vi "Configure_Voltage.vi"(8 "error in (no error)":errorcluster, 10 "DC_Voltage_Configuration":variant, 11 "NI-DMM in":refnum<class "NI-DCPower.lvclass">) -> (0 "error out":errorcluster, 3 "NI-DMM out":refnum<class "NI-DCPower.lvclass">)   [LabVIEW 2020, in "NI-DCPower.lvclass"]
uses:
  NI-DCPower.lvclass
  C:/Program Files/National Instruments/LabVIEW 2020/vi.lib/MeasurementLink/MeasurementLink Instrument/ISession Factory/ISession Factory.lvclass
  Typedefs/Configure_Parameters.ctl
  <vilib>/MeasurementLink/MeasurementLink Session Management V1/Session Reservation/Pin Type.ctl
  Typedefs/connection with session.ctl
  <vilib>/MeasurementLink/MeasurementLink Session Management V1/Session Reservation/Connection.ctl
  <instrlib>/niDCPower/nidcpower.llb/niDCPower Source Mode.ctl
  f01df658-2e31-4a97-abfd-bc2b634ba6ad.vi
  <vilib>/MeasurementLink/MeasurementLink Session Management V1/Session Reservation/Get Connections Impl.vi
  <vilib>/MeasurementLink/MeasurementLink Session Management V1/Session Reservation/Session Reservation.lvclass
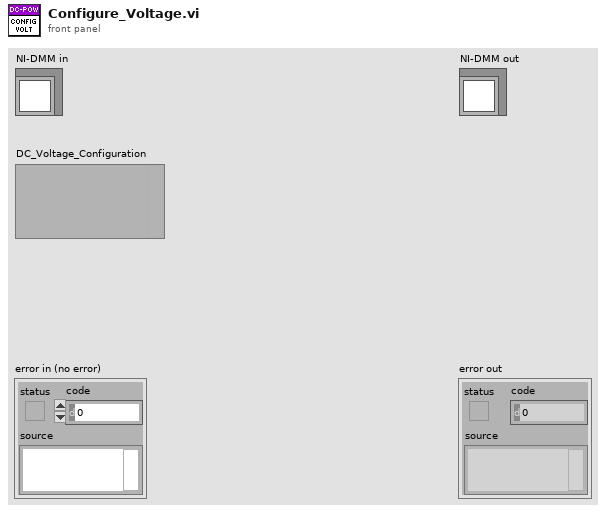
[diagram p1: front panel]
types:
  T1 = typedef "NI-DCPower.lvclass/connection with session.ctl" = cluster{"connection":T2, "session":refnum<k15>}
  T2 = typedef "MeasurementLink Session Management V1.lvlib/Session Reservation.lvclass/Connection.ctl" = cluster{"pin or relay name":string, "site":i32, "instrument type id":string, "channel":string}
  T3 = typedef "MeasurementLink Session Management V1.lvlib/Session Reservation.lvclass/Pin Type.ctl" = enum16{"DUT and System Pins", "System Pins"}
  T4 = typedef "NI-DCPower.lvclass/Configure_Parameters.ctl" = cluster{"pin name":string[], "Range":dbl, "Measurement Type":enum32{"DC Volts", "AC Volts", "DC Current", "AC Current", "2-wire Resistance", "4-wire Resistance", "Diode", "Frequency", "Period", "AC Volts DC Coupled", "Capacitance", "Inductance", "Temperature"}, "Resolution in Digits":enum32{"3 1/2", "4 1/2", "5 1/2", "6 1/2", "7 1/2"}}
  T5 = enum32{"DC Volts", "AC Volts", "DC Current", "AC Current", "2-wire Resistance", "4-wire Resistance", "Diode", "Frequency", "Period", "AC Volts DC Coupled", "Capacitance", "Inductance", "Temperature"}
  T6 = typedef "niDCPower Source Mode.ctl" = i32
  T7 = typedef "niDCPower Output Function.ctl" = i32
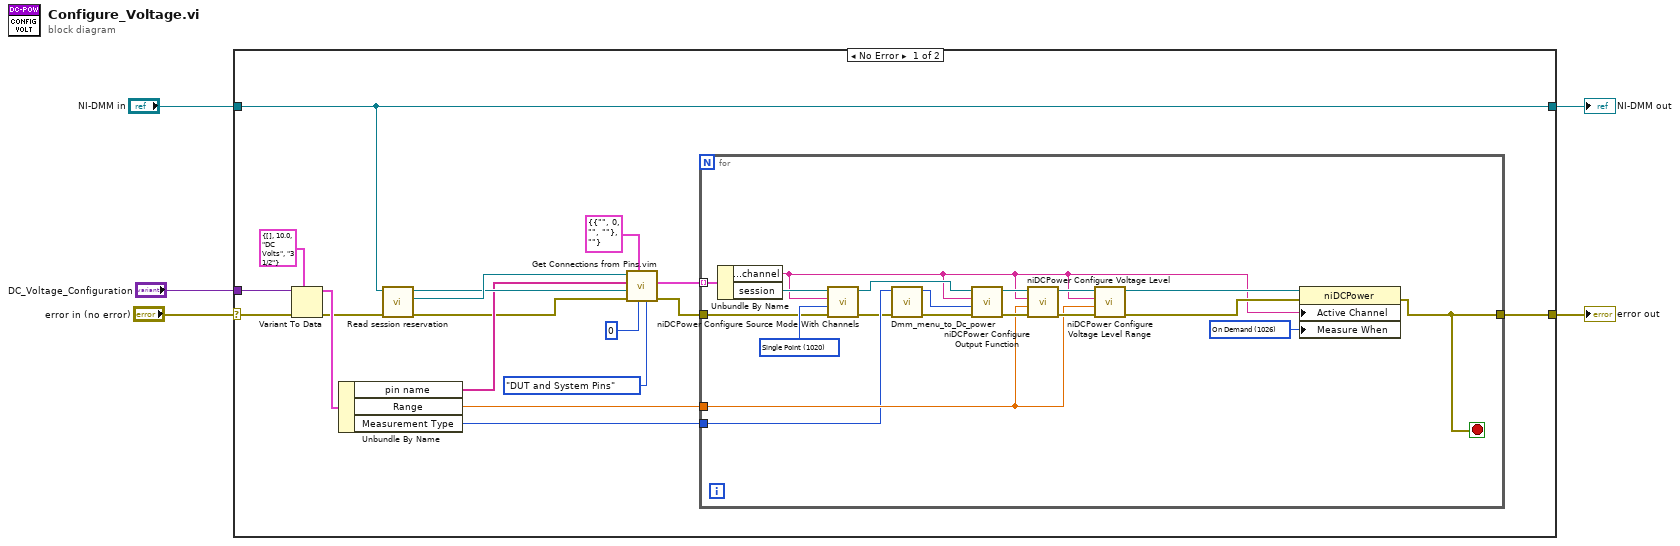
[diagram p0: block diagram]
diagram:
  n1 = case shown="No Error" "error in (no error)" {
    selector: "error in (no error)" -> [w23 w43]
    tunnel: "DC_Voltage_Configuration" -> [w22 _]
    tunnel: [w18 w43] -> w3
    tunnel: "NI-DMM in" -> [w14 w44]
    tunnel: [w14 w44] -> w1
    frame No Error {
      n2 = Variant To Data(error in=w23, type=T4 {"pin name"=[], "Range"=10.0, "Measurement Type"=enum."DC Volts", "Resolution in Digits"=enum."3 1/2"}, Variant=w22) -> (data=w20:T4, error out=w17:errorcluster)
      n3 = Unbundle By Name(w20) -> ("pin name"=w11:string[], "Range"=w19:dbl, "Measurement Type"=w6:T5)
      n4 = call-dynamic "Read session reservation.vi"("error in (no error)"=w17, "Abstract_Instrument in"=w14) -> ("error out"=w10:errorcluster, "Session Reservation.lvclass"=w13:refnum<class "Session Reservation.lvclass">, "Abstract_Instrument out"=w12:refnum<class "NI-DCPower.lvclass">)  [unwired: 7 in]
      n5 = call "Get Connections from Pins.vim"("pin type"=Pin_Type."DUT and System Pins", "site"=0, "connection type"=T1 {"connection"={"pin or relay name"="", "site"=0, "instrument type id"="", "channel"=""}, "session"=""} ("connection with session"), "error in"=w10, "session factory"=w12, "pin or relay names"=w11, "session reservation in"=w13) -> ("error out"=w9:errorcluster, "connections"=w7:T1[])  [unwired: 2 in, 1 out]
      n6 = for {
        tunnel: w19 -> [w28]
        tunnel: [w30] -> w18
        tunnel: w9 -> [w33]
        tunnel: w7 -> [w42] mode=indexing
        tunnel: w6 -> [w26]
        stop <- w30 stop-if-true
        w29 = 1026 items=["Automatically after Source Complete"=1025, "On Demand"=1026, "On Measure Trigger"=1027] ("Measurement:Advanced:Measure When")
        w34 = T6 1020 items=["Single Point"=1020, "Sequence"=1021] ("source mode")
        n7 = Unbundle By Name(w42) -> ("connection.channel"=w31:string, "session"=w32:refnum<k15>)
        n8 = call <instrlib>:"niDCPower Configure Source Mode With Channels.vi"("error in (no error)"=w33, "source mode"=w34, "channel name"=w31, "instrument handle"=w32) -> ("error out"=w25:errorcluster, "instrument handle out"=w39:refnum<k15>)  [unwired: 6 in]
        n9 = call "Dmm_menu_to_Dc_power.vi"("error in (no error)"=w25, "Measurement Type"=w26) -> ("error out"=w24:errorcluster, "output function"=w27:T7)  [unwired: 8 in]
        n10 = call <instrlib>:"niDCPower Configure Output Function.vi"("error in (no error)"=w24, "output function"=w27, "channel name"=w31, "instrument handle"=w39) -> ("error out"=w35:errorcluster, "instrument handle out"=w36:refnum<k15>)  [unwired: 6 out]
        n11 = call <instrlib>:"niDCPower Configure Voltage Level.vi"("error in (no error)"=w35, "voltage level"=w28, "channel name"=w31, "instrument handle"=w36) -> ("error out"=w40:errorcluster, "instrument handle out"=w41:refnum<k15>)  [unwired: 6 out]
        n12 = call <instrlib>:"niDCPower Configure Voltage Level Range.vi"("error in (no error)"=w40, "voltage level range"=w28, "channel name"=w31, "instrument handle"=w41) -> ("error out"=w38:errorcluster, "instrument handle out"=w37:refnum<k15>)  [unwired: 6 out]
        n13 = property class="niDCPower"(reference=w37, error in=w38, "Active Channel"=w31, "Measure When"=w29) -> (error out=w30:errorcluster)  [unwired: 1 out]
      }
    }
    frame Error {
    }
  }
  "error out" <- w3
  "NI-DMM out" <- w1
